vi "temp_huniditydht11_niusb6009.vi"() -> ()   [LabVIEW 2020]
panel:
  out "Waveform Chart":dynamicdata(graph)
  in  "stop":bool
  out "Numeric":dbl
  out "temperature 0 C":dynamicdata(graph)
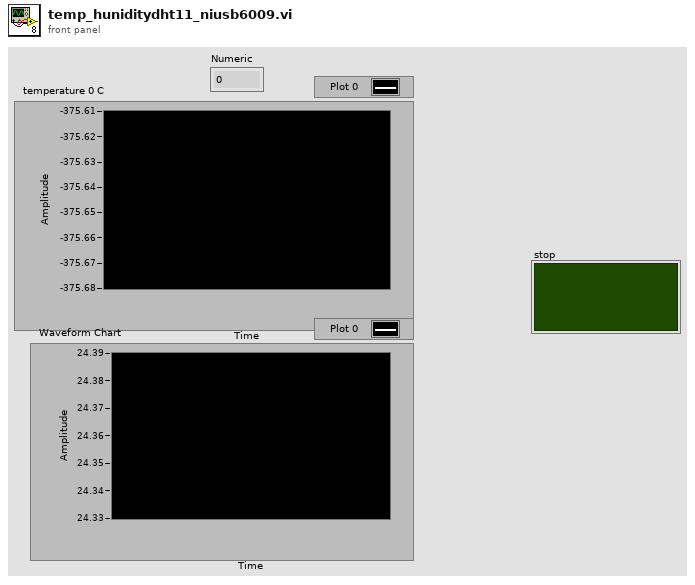
[diagram p1: front panel]
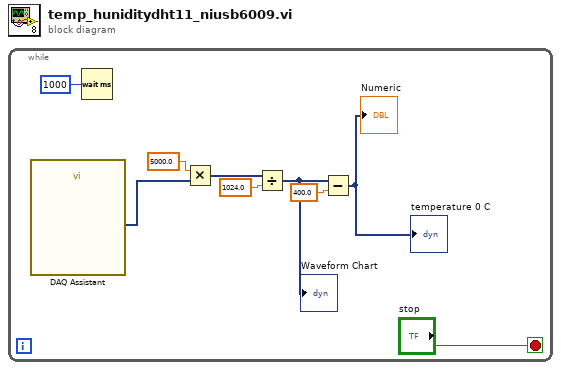
[diagram p0: block diagram]
diagram:
  n1 = while {
    stop <- "stop" stop-if-true
    n2 = call "DAQ Assistant"() -> ("data"=w8:dynamicdata)  [unwired: 17 in, 2 out]
    n3 = Wait (ms)(milliseconds to wait=u32 1000) -> ()  [unwired: 1 out]
    n4 = Multiply(x=5000.0, y=w8) -> (x*y=w6:dynamicdata)
    n5 = Divide(x=w6, y=1024.0) -> (x/y=w1:dynamicdata)
    "Waveform Chart" <- w1
    n6 = Subtract(x=w1, y=400.0) -> (x-y=→"temperature 0 C" →"Numeric":dynamicdata)
  }
